vi "900x 9870 Interrupt Config (Sub).vi"(5 "EOS Byte":u8=10, 7 "Enable EOS":bool=TRUE, 8 "error in":errorcluster, 10 "Byte Timeout":i32=100, 11 "FPGA In":T1) -> (0 "error out":errorcluster, 3 "FPGA Out":T1)   [LabVIEW 2012]
uses:
  900x INT FPGA Reference.ctl
  <vilib>/Utility/error.llb/Error Cluster From Error Code.vi
  <vilib>/rvi/errors/niLvFpgaAdjustHostInterfaceError.vi
  <vilib>/rvi/interface/nirviReadWriteControl/nirviReadWriteControl.xnode
  FPGA Bitfiles/NI-987xSerialLoo_FPGATarget3_9870InterfaceInt_BB93BC1A.lvbitx
  Program Files (x86)/National Instruments/LabVIEW 2012/examples/CompactRIO/Module Specific/NI 987x/Serial Loopback/VIs/9870 Interface Interrupt (FPGA).vi
  NiFpgaLv.dll
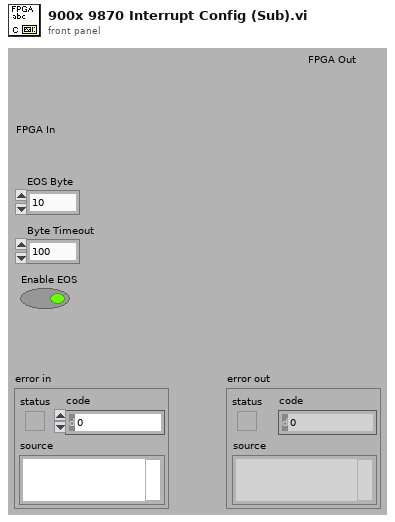
[diagram p1: front panel]
types:
  T1 = typedef "900x INT FPGA Reference.ctl" = refnum<k20>
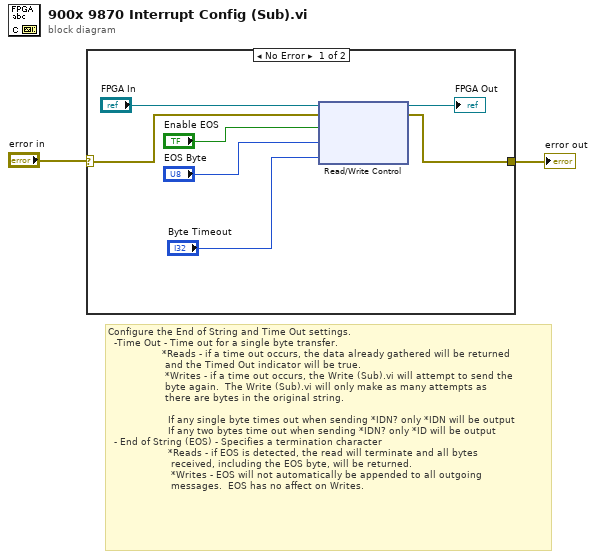
[diagram p0: block diagram]
diagram:
  # "Configure the End of String and Time Out settings.  \n  -Time Out - Time out for a single byte transfer.\n                  *Reads - if a time out occurs, the data already gathered will be returned\n                   and the Timed Out indicator will be true.\n                   *Writes - if a time out occurs, the Write (Sub).vi will attempt to send the \n                   byte again.  The Write (Sub).vi will only make as many attempts as \n                   there are bytes in the original string.\n                   \n                    If any single byte times out when sending *IDN? only *IDN will be output\n                    If any two bytes time out when sending *IDN? only *ID will be output\n  - End of String (EOS) - Specifies a termination character\n                    *Reads - if EOS is detected, the read will terminate and all bytes \n                     received, including the EOS byte, will be returned.\n                     *Writes - EOS will not automatically be appended to all outgoing \n                     messages.  EOS has no affect on Writes."
  n1 = case shown="No Error" "error in" {
    selector: "error in" -> [w4 w10]
    tunnel: [w3 w10] -> w1
    frame No Error {
      n2 = xnode "Read/Write Control"("FPGA VI Reference In"="FPGA In", "error in"=w4, "EOS Enabled"="Enable EOS", "EOS"="EOS Byte", "Byte Timeout"="Byte Timeout") -> ("FPGA VI Reference Out"=→"FPGA Out":T1, "error out"=w3:errorcluster)
    }
    frame Error {
    }
  }
  "error out" <- w1
